vi "Rs232_Read-v3.vi"() -> ()   [LabVIEW 2020]
uses:
  <vilib>/Instr/_visa.llb/VISA Configure Serial Port (Instr).vi
panel:
  out "read buffer (Number)":dbl
  out "Waveform Chart":dbl(graph)
  in  "stop":bool
  out "error out":errorcluster
  out "read buffer (String)":string
  in  "VISA resource name":refnum<visa-resource-name>
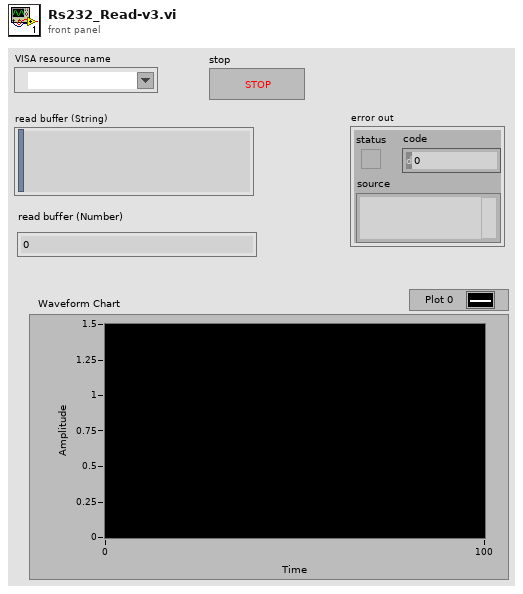
[diagram p1: front panel]
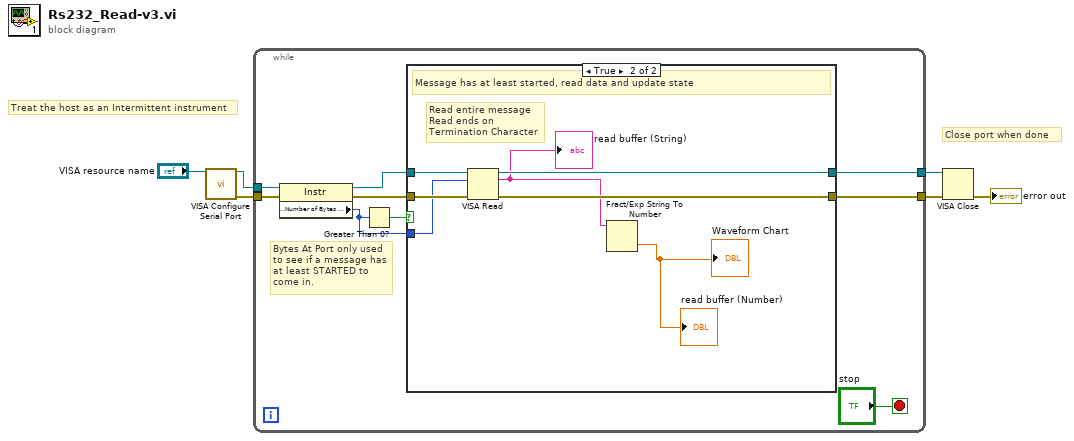
[diagram p0: block diagram]
diagram:
  # "Treat the host as an Intermittent instrument"
  # "Close port when done"
  n1 = call-poly "VISA Configure Serial Port"("VISA resource name"="VISA resource name") -> ("VISA resource name out"=w1:refnum<visa-resource-name>, "error out"=w4:errorcluster)  [unwired: 13 in]
  n2 = while {
    tunnel: w4 -> [w15]
    tunnel: w1 -> [w12]
    tunnel: [w9] -> w2
    tunnel: [w13] -> w6
    stop <- "stop" stop-if-true
    # "Bytes At Port only used\nto see if a message has\nat least STARTED to\ncome in."
    n3 = property class="Instr"(reference=w12, error in=w15) -> (reference out=w10:refnum<visa-resource-name>, error out=w14:errorcluster, "Serial Settings:Number of Bytes at Serial Port"=w7:u32)
    n4 = Greater Than 0?(x=w7) -> (x > 0?=w11:bool)
    n5 = case shown="True" w11 {
      tunnel: w14 -> [w16 w24]
      tunnel: w10 -> [w17 w22]
      tunnel: [w17 w21] -> w9
      tunnel: [w16 w23] -> w13
      tunnel: w7 -> [_ w20]
      frame False {
        # "No message.  If enough time has passed, send new measurement"
      }
      frame True {
        # "Read entire message\nRead ends on\nTermination Character"
        # "Message has at least started, read data and update state"
        n6 = VISA Read(VISA resource name=w22, byte count=w20, error in (no error)=w24) -> (VISA resource name out=w21:refnum<visa-resource-name>, read buffer=w19:string, error out=w23:errorcluster)  [unwired: 1 out]
        "read buffer (String)" <- w19
        n7 = Fract/Exp String To Number(string=w19) -> (number=→"Waveform Chart" →"read buffer (Number)":dbl)  [unwired: 3 in, 1 out]
      }
    }
  }
  n8 = VISA Close(VISA resource name=w2, error in (no error)=w6) -> (error out=→"error out":errorcluster)
